vi "writeOutDcamImg.vi"(1 "stackFname":path=path "C:/Users/sims01/Desktop/dataAcq", 2 "sCMOShandle":u32) -> (0 "stackComplete":bool)   [LabVIEW 2015]
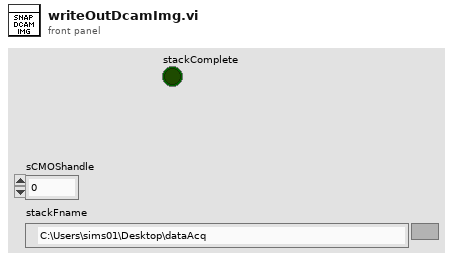
[diagram p1: front panel]
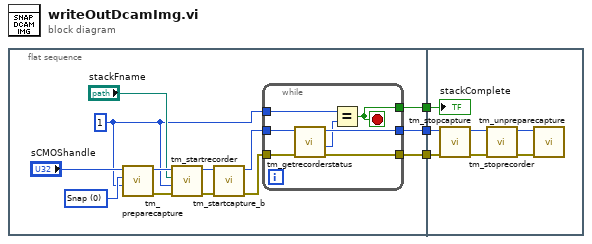
[diagram p0: block diagram]
diagram:
  n1 = flat-sequence {
    tunnel: [w6] -> w3
    tunnel: [w5] -> w2
    tunnel: [w4] -> w1
    tunnel: w3 -> [w26]
    tunnel: w2 -> [w25]
    tunnel: w1 -> [w24]
    frame #0 {
      w7 = 1 ("Frames")
      w15 = 0 items=["Snap", "Sequence"] ("Capture mode")
      n2 = call <userlib>:"tm_preparecapture.vi"("Frames"=w7, "Capture mode"=w15, "Handle in"="sCMOShandle") -> ("error out"=w13:errorcluster, "Handle out"=w16:u32)  [unwired: 5 in, 2 out]
      n3 = call <userlib>:"tm_startrecorder.vi"("error in (no error)"=w13, "frames"=w7, "File"="stackFname", "Handle in"=w16) -> ("error out"=w12:errorcluster, "Handle out"=w14:u32)  [unwired: 6 in]
      n4 = call <userlib>:"tm_startcapture_b.vi"("error in (no error)"=w12, "Handle in"=w14) -> ("error out"=w8:errorcluster, "Handle out"=w9:u32)  [unwired: 8 in]
      n5 = while {
        tunnel: w9 -> [w23]
        tunnel: w8 -> [w22]
        tunnel: w7 -> [w17]
        tunnel: [w21] -> w6
        tunnel: [w20] -> w5
        tunnel: [w19] -> w4
        stop <- w21 stop-if-true
        n6 = call <userlib>:"tm_getrecorderstatus.vi"("error in (no error)"=w22, "Handle"=w23) -> ("error out"=w19:errorcluster, "Count"=w18:i32, "Handle"=w20:u32)  [unwired: 6 in, 1 out]
        n7 = Equal?(x=w17, y=w18) -> (x = y?=w21:bool)
      }
    }
    frame #1 {
      n8 = call <userlib>:"tm_stopcapture.vi"("error in (no error)"=w24, "Handle in"=w25) -> ("error out"=w28:errorcluster, "Handle out"=w27:u32)  [unwired: 8 in]
      n9 = call <userlib>:"tm_stoprecorder.vi"("error in (no error)"=w28, "Handle in"=w27) -> ("error out"=w29:errorcluster, "Handle out"=w30:u32)  [unwired: 8 in]
      n10 = call <userlib>:"tm_unpreparecapture.vi"("error in (no error)"=w29, "Handle in"=w30) -> ()  [unwired: 8 in, 2 out]
      "stackComplete" <- w26
    }
  }
